vi "Utility Factory Reset.vi"(7 "Retry Attempts (0)":i32 min=0, 8 "error in (no error)":errorcluster, 11 "VISA resource name":refnum<visa-resource-name>) -> (0 "error out":errorcluster, 3 "VISA resource name out":refnum<visa-resource-name>)   [LabVIEW 2020, in "Omega Platinum Series.lvlib"]
doc: "Resets the instrument and then sends a set of default setup commands to the instrument."
uses:
  Omega Platinum Series.lvlib
panel:
  # "USE WITH EXTREME CAUTION, WILL CAUSE FACTORY RESET"
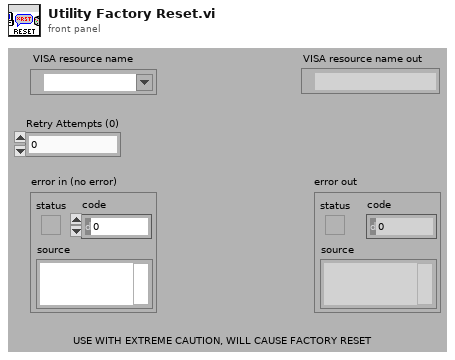
[diagram p1: front panel]
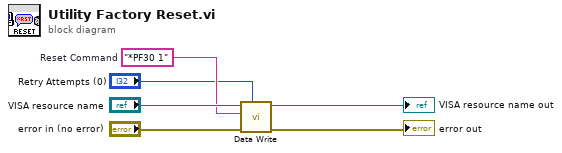
[diagram p0: block diagram]
diagram:
  w2 = "*PF30 1"  # Reset Command
  n1 = call "Data Write.vi"("Retry Attempts (0)"="Retry Attempts (0)", "error in (no error)"="error in (no error)", "Command"=w2, "VISA Refnum in"="VISA resource name") -> ("error out"=→"error out":errorcluster, "VISA Refnum out"=→"VISA resource name out":refnum<visa-resource-name>)  [unwired: 6 in]
